vi "Get Calibrated Amplitude per Site.vi"(0 "TSM context":T1, 5 "dB SPL":dbl, 7 "Frequency (Hz)":dbl, 11 "error in (no error)":errorcluster) -> (4 "Per Site Amplitude (V)":dbl[](array[numeric]), 6 "Found?":bool, 15 "error out":errorcluster)   [LabVIEW 2020]
doc: "Gets the required Amplitude(V) for the given dB SPL - Frequency(Hz) pair for each site"
uses:
  <vilib>/NI_TestStand_SemiconductorModule/NI_TestStand_Semiconductor_Module.lvlibp/PinMap/General/SemiconductorModuleContext.ctl
  8aa3e1a0-ac19-45a6-a176-8639637103f1.vi
  8aa3e1a0-ac19-45a6-a176-8639637103f1.vi/5af0aee7-fadd-4518-80df-464b05248f55.vi
  <vilib>/gmath/interp.llb/Interpolate 2D.vi
  <vilib>/gmath/interp.llb/Interpolate 2D (1d xi,yi).vi
  <vilib>/Utility/error.llb/Error Cluster From Error Code.vi
  <vilib>/NI_TestStand_SemiconductorModule/NI_TestStand_Semiconductor_Module.lvlibp
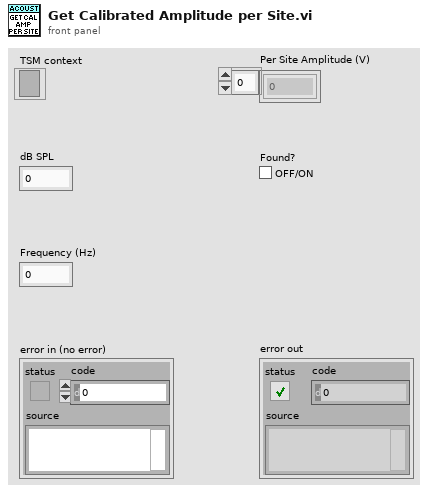
[diagram p1: front panel]
types:
  T1 = typedef "NI_TestStand_Semiconductor_Module.lvlibp/SemiconductorModuleContext.ctl" = refnum<k7>
  T2 = typedef "Acoustic Cal Data Cluster.ctl" = cluster{"Site Number":i32, "Serial Number":u32, "Ref Mic Sensitivity":dbl, "SPL Axis":dbl[], "Frequency Axis":dbl[], "Speaker Vp":dbl[][], "Ref Mic Cal File Data":string[][], "Speaker Vp Axis":dbl[], "SPL Measurements":dbl[][]}
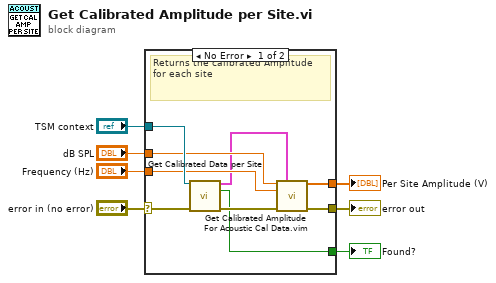
[diagram p0: block diagram]
diagram:
  n1 = case shown="No Error" "error in (no error)" {
    selector: "error in (no error)" -> [w15 w17]
    tunnel: "TSM context" -> [w16 _]
    tunnel: "dB SPL" -> [w14 _]
    tunnel: "Frequency (Hz)" -> [w13 _]
    tunnel: [w11 _] -> w1
    tunnel: [w10 w17] -> w3
    tunnel: [w9 _] -> w2
    frame No Error {
      # "Returns the calibrated Amplitude for each site"
      n2 = call "Get Calibrated Data per Site.vi"("TSM context"=w16, "error in (no error)"=w15) -> ("Per Site Acoustic Cal Data"=w8:T2[], "Found?"=w9:bool, "error out"=w12:errorcluster)  [unwired: 11 in]
      n3 = call "Get Calibrated Amplitude For Acoustic Cal Data.vim"("dB SPL"=w14, "Acoustic Cal Data"=w8, "Frequency"=w13, "error in (no error)"=w12) -> ("Amplitude"=w11:dbl[], "error out"=w10:errorcluster)  [unwired: 10 in]
    }
    frame Error {
      # "Error - Do Nothing"
    }
  }
  "error out" <- w3
  "Found?" <- w2
  "Per Site Amplitude (V)" <- w1
